vi "NF WF1973_74 TRIG Slop.vi"(6 "Read(F)":bool, 7 "Set(Sweep)":bool, 8 "error in (no error)":errorcluster caption="Error IN", 9 "Slope(Positive)":u32(ring) items=["Positive", "Negative", "OFF"], 10 "Channel(Ch1)":bool, 11 "VISAsession":refnum<visa-resource-name>) -> (0 "error out":errorcluster caption="Error OUT", 2 "Query Slope":string, 3 "CopyVISAsession":refnum<visa-resource-name>)   [LabVIEW 2010]
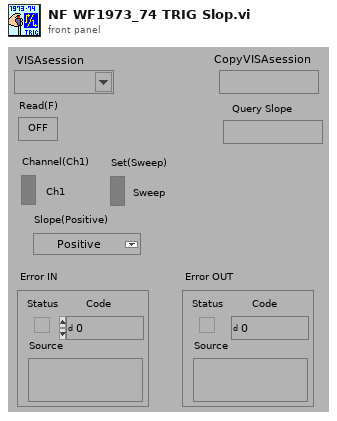
[diagram p1: front panel]
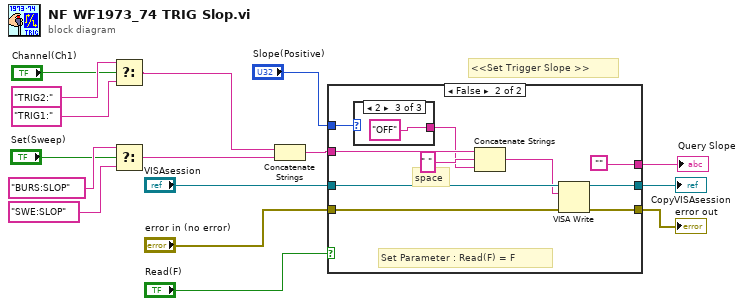
[diagram p0: block diagram]
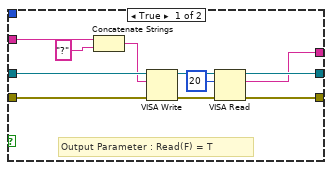
[diagram p2: hidden frame]
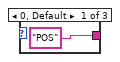
[diagram p3: hidden frame]
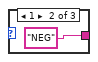
[diagram p4: hidden frame]
diagram:
  # "<<Set Trigger Slope >>"
  n1 = Select(t="TRIG2:" ("文字列"), s="Channel(Ch1)", f="TRIG1:" ("文字列")) -> (s? t:f=w2:string)
  n2 = Select(t="BURS:SLOP", s="Set(Sweep)", f="SWE:SLOP") -> (s? t:f=w1:string)
  n3 = Concatenate Strings(w2, w1) -> (w4:string)
  n4 = case shown="FALSE" "Read(F)" {
    tunnel: "VISAsession" -> [w27 w37]
    tunnel: [w24 w35] -> w15
    tunnel: [w23 w36] -> w14
    tunnel: "error in (no error)" -> [w22 w29]
    tunnel: w4 -> [w20 w32]
    tunnel: "Slope(Positive)" -> [_ w31]
    tunnel: [w17 ""] -> w10
    frame True {
      # "Output Parameter : Read(F) = T"
      n5 = Concatenate Strings(w20, "?" ("形式文字列")) -> (w18:string)
      n6 = VISA Write(VISA resource name=w27, write buffer=w18, error in (no error)=w22) -> (VISA resource name out=w25:refnum<visa-resource-name>, error out=w26:errorcluster)  [unwired: 1 out]
      n7 = VISA Read(VISA resource name=w25, byte count=u32 20 ("バイトカウント（0）"), error in (no error)=w26) -> (VISA resource name out=w24:refnum<visa-resource-name>, read buffer=w17:string, error out=w23:errorcluster)  [unwired: 1 out]
    }
    frame False {
      # "space"
      # "Set Parameter : Read(F) = F"
      n8 = case shown="2" w31 {
        tunnel: ["POS" "NEG" "OFF"] -> w30
        frame 0, Default {
        }
        frame 1 {
        }
        frame 2 {
        }
      }
      n9 = Concatenate Strings(w32, " ", w30) -> (w34:string)
      n10 = VISA Write(VISA resource name=w37, write buffer=w34, error in (no error)=w29) -> (VISA resource name out=w35:refnum<visa-resource-name>, error out=w36:errorcluster)  [unwired: 1 out]
    }
  }
  "error out" <- w14
  "CopyVISAsession" <- w15
  "Query Slope" <- w10
